vi "CheckAndRefresh.vi"(8 "error in (no error)":errorcluster, 11 "ControlState in":T1 {"ChainMask" format="0x%02x"}) -> (0 "error out":errorcluster, 3 "ControlState out":T1 {"ChainMask" format="0x%02x"})   [LabVIEW 2018, in "ArduinoSerialBling.lvlib"]
uses:
  ArduinoSerialBling.lvlib
  ControlState.ctl
  ConnectionType.ctl
  UdpConnection.ctl
  ChainState.ctl
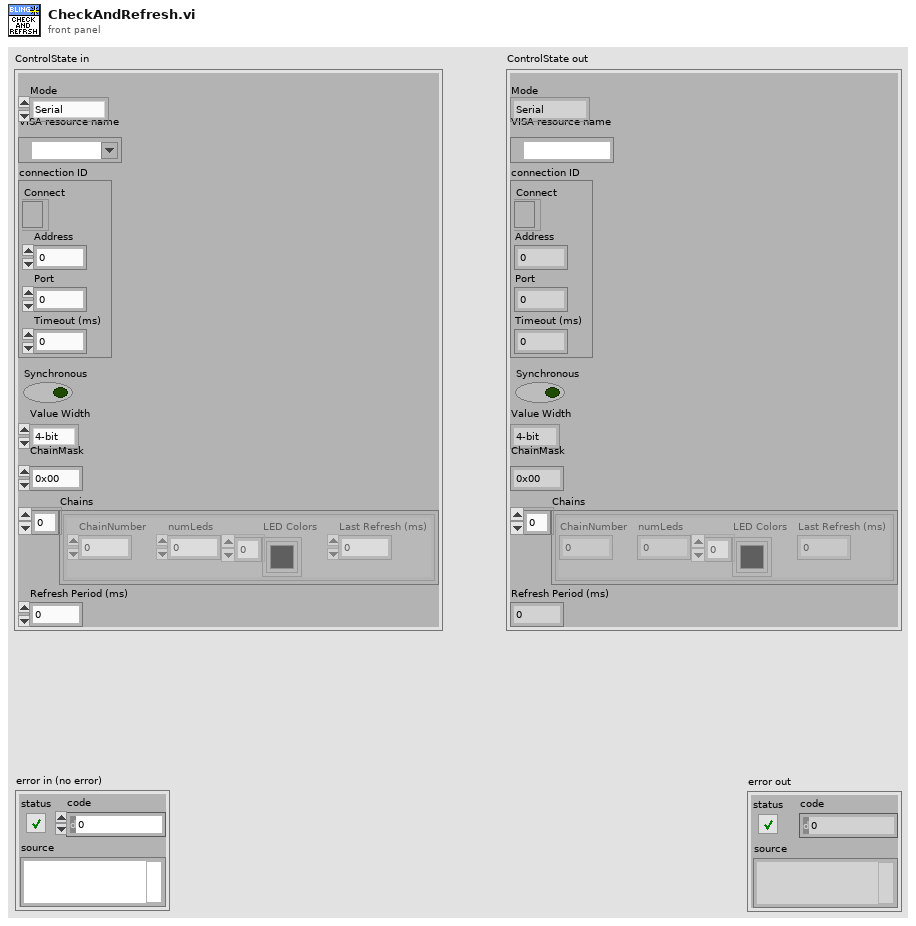
[diagram p1: front panel]
types:
  T1 = typedef "ArduinoSerialBling.lvlib/ControlState.ctl" = cluster{"Mode":T2, "VISA resource name":refnum<visa-resource-name>, "connection ID":T3, "Synchronous":bool, "Value Width":enum16{"4-bit", "8-bit"}, "ChainMask":u8, "Chains":T4[], "Refresh Period (ms)":u32}
  T2 = typedef "ConnectionType.ctl" = enum16{"Serial", "Ethernet", "Offline"}
  T3 = typedef "UdpConnection.ctl" = cluster{"Connect":refnum<k16>, "Address":u32, "Port":u16, "Timeout (ms)":i32}
  T4 = typedef "ArduinoSerialBling.lvlib/ChainState.ctl" = cluster{"ChainNumber":u8, "numLeds":u8, "LED Colors":u32[], "Last Refresh (ms)":u32}
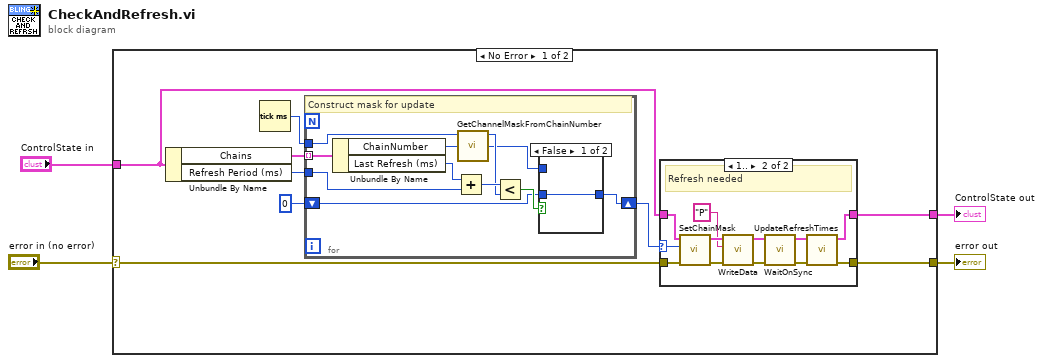
[diagram p0: block diagram]
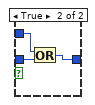
[diagram p3: hidden frame]
diagram:
  n1 = case shown="No Error" "error in (no error)" {
    selector: "error in (no error)" -> [w8 w42]
    tunnel: [w7 w43] -> w3
    tunnel: "ControlState in" -> [w9 w43]
    tunnel: [w6 w42] -> w1
    frame No Error {
      n2 = Unbundle By Name(w9) -> ("Chains"=w13:T4[], "Refresh Period (ms)"=w12:u32)
      n3 = Tick Count (ms)() -> (millisecond timer value=w11:u32)
      n4 = for {
        tunnel: w13 -> [w37] mode=indexing
        tunnel: w12 -> [w35]
        tunnel: w11 -> [w33]
        shift-right: [w28] -> w5
        shift-left: u8 0 -> [w29]
        # "Construct mask for update"
        n5 = Unbundle By Name(w37) -> ("ChainNumber"=w32:u8, "Last Refresh (ms)"=w36:u32)
        n6 = Add(x=w36, y=w35) -> (x+y=w34:u32)
        n7 = call "GetChannelMaskFromChainNumber.vi"("ChainNumber"=w32) -> ("ChainMask"=w30:u8)
        n8 = Less?(x=w34, y=w33) -> (x < y?=w31:bool)
        n9 = case shown="False" w31 {
          tunnel: w30 -> [_ w41]
          tunnel: w29 -> [w38 w40]
          tunnel: [w38 w39] -> w28
          frame False {
          }
          frame True {
            n10 = Or(x=w41, y=w40) -> (x .or. y?=w39:u8)
          }
        }
      }
      n11 = case shown="1.." w5 {
        selector: w5 -> [_ w16]
        tunnel: w9 -> [w14 w27]
        tunnel: w8 -> [w15 w26]
        tunnel: [w14 w18] -> w7
        tunnel: [w15 w17] -> w6
        frame 0, Default {
          # "No refresh needed"
        }
        frame 1.. {
          # "Refresh needed"
          n12 = call "SetChainMask.vi"("error in (no error)"=w26, "ChainMask"=w16, "ControlState in"=w27) -> ("error out"=w23:errorcluster, "ControlState out"=w25:T1)  [unwired: 7 in]
          n13 = call "WriteData.vi"("error in (no error)"=w23, "Command"="P", "ControlState in"=w25) -> ("error out"=w21:errorcluster, "ControlState out"=w22:T1)  [unwired: 5 in, 2 out]
          n14 = call "WaitOnSync.vi"("error in (no error)"=w21, "ControlState in"=w22) -> ("error out"=w20:errorcluster, "ControlState out"=w19:T1)  [unwired: 8 in]
          n15 = call "UpdateRefreshTimes.vi"("error in (no error)"=w20, "ControlState in"=w19) -> ("error out"=w17:errorcluster, "ControlState out"=w18:T1)  [unwired: 8 in]
        }
      }
    }
    frame Error {
    }
  }
  "error out" <- w1
  "ControlState out" <- w3
